vi "JKI.Robot.SMO.TestUI.TestLauncher.vi"() -> ()   [LabVIEW 2014, in "JKI.Robot.SMO.APITesterUI.lvclass"]
doc: "JKI State Machine Objects (SMO) 1.0.0.5\nJKI - JKI\nCopyright (c) 2016, JKI"
uses:
  JKI.Robot.SMO.APITesterUI.lvclass
  <vilib>/JKI/JKI SMO/SMO/SMO.lvclass
  <vilib>/JKI/JKI SMO/SMO.UI/SMO.UI.lvclass
panel:
  out "error out":errorcluster
  in  "Stop":bool
  # "SMO UI Test Launcher"
  # "For instructions on how to use the JKI State Machine Objects, examples and video tutorials, visit:\nhttp://jki.net/state-machine-objects/\n\nJKI State Machine Objects™\nhttp://jki.net/state-machine-objects/\nCopyright (C) 2005-2015, JKI <info@jki.net>\nALL RIGHTS RESERVED"
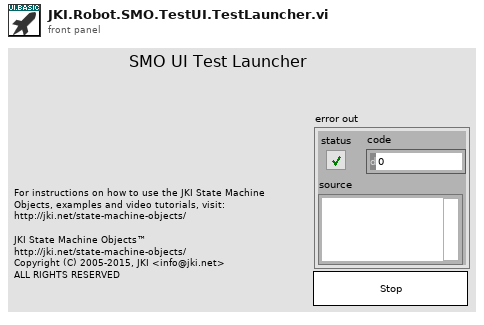
[diagram p1: front panel]
types:
  T1 = typedef "SMO.UI.lvclass/PublicEvents--Cluster.ctl" = cluster{"UI Hidden":refnum<user-event>, "UI State":refnum<user-event>}
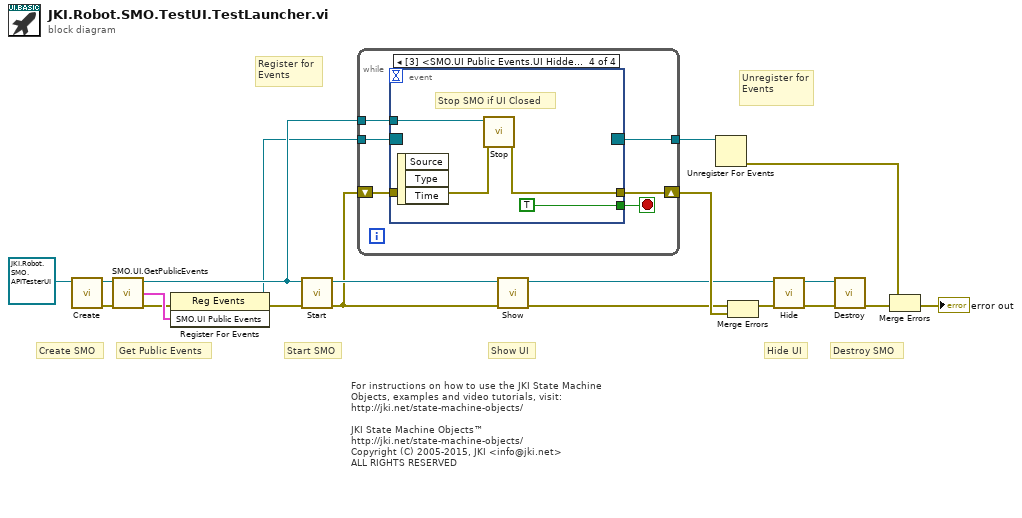
[diagram p0: block diagram]
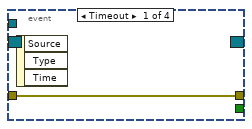
[diagram p2: hidden frame]
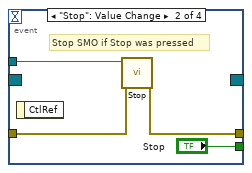
[diagram p3: hidden frame]
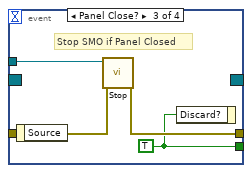
[diagram p4: hidden frame]
diagram:
  # "Hide UI"
  # "Show UI"
  # "For instructions on how to use the JKI State Machine Objects, examples and video tutorials, visit:\nhttp://jki.net/state-machine-objects/\n\nJKI State Machine Objects™\nhttp://jki.net/state-machine-objects/\nCopyright (C) 2005-2015, JKI <info@jki.net>\nALL RIGHTS RESERVED"
  # "Get Public Events"
  # "Start SMO"
  # "Destroy SMO"
  # "Create SMO"
  # "Unregister for Events"
  # "Register for Events"
  n1 = call <vilib>:"Create.vi"("SMO"=refnum<class "JKI.Robot.SMO.APITesterUI.lvclass"> refnum ("SMO.Template.lvclass")) -> ("error out"=w6:errorcluster, "SMO out"=w7:refnum<class "JKI.Robot.SMO.APITesterUI.lvclass">)  [unwired: 8 in, 1 out]
  n2 = call <vilib>:"SMO.UI.GetPublicEvents.vi"("error in (no error)"=w6, "SMO.UI"=w7) -> ("error out"=w3:errorcluster, "SMO.UI Public Events"=w4:T1, "SMO.UI out"=w5:refnum<class "JKI.Robot.SMO.APITesterUI.lvclass">)  [unwired: 7 in]
  n3 = register-events(error in=w3, w4) -> (reference out=w1:refnum<event-registration>, error out=w2:errorcluster)  [unwired: 1 in]
  n4 = call <vilib>:"Start.vi"("error in (no error)"=w2, "SMO"=w5) -> ("error out"=w13:errorcluster, "SMO out"=w14:refnum<class "JKI.Robot.SMO.APITesterUI.lvclass">)  [unwired: 8 in]
  n5 = while {
    shift-right: [w25] -> w19
    shift-left: w13 -> [w24]
    tunnel: w1 -> [w23]
    tunnel: [w22] -> w20
    tunnel: w5 -> [w21]
    stop <- w26 stop-if-true
    n6 = event shown="[3] <SMO.UI Public Events.UI Hidden>: User Event" {
      selector: w23 -> [_ _ _ _]
      dyn-events: [_ _ _ _] -> w22
      timeout: _ -> [_ _ _ _]
      tunnel: [_ "Stop" w32 TRUE ("OK")] -> w26
      tunnel: w21 -> [_ w29 w35 w39]
      tunnel: [w27 w30 w34 w38] -> w25
      tunnel: w24 -> [w27 w28 w33 w37]
      event Timeout {
        n7 = event-data() -> ()  [unwired: 1 in, 3 out]
      }
      event "Stop": Value Change {
        # "Stop SMO if Stop was pressed"
        n8 = event-data() -> ()  [unwired: 1 in, 1 out]
        n9 = call <vilib>:"Stop.vi"("error in (no error)"=w28, "SMO"=w29) -> ("error out"=w30:errorcluster)  [unwired: 8 in, 1 out]
      }
      event Panel Close? {
        w32 = TRUE ("OK")
        # "Stop SMO if Panel Closed"
        n10 = event-data() -> ()  [unwired: 1 in, 1 out]
        n11 = call <vilib>:"Stop.vi"("error in (no error)"=w33, "SMO"=w35) -> ("error out"=w34:errorcluster)  [unwired: 8 in, 1 out]
        n12 = event-data("Discard?"=w32) -> ()  [unwired: 1 in, 1 out]
      }
      event User Event {
        # "Stop SMO if UI Closed"
        n13 = event-data() -> ()  [unwired: 1 in, 3 out]
        n14 = call <vilib>:"Stop.vi"("error in (no error)"=w37, "SMO"=w39) -> ("error out"=w38:errorcluster)  [unwired: 8 in, 1 out]
      }
    }
  }
  n15 = call <vilib>:"Show.vi"("error in (no error)"=w13, "SMO.UI"=w14) -> ("error out"=w12:errorcluster, "SMO.UI out"=w11:refnum<class "JKI.Robot.SMO.APITesterUI.lvclass">)  [unwired: 8 in]
  n16 = Unregister For Events(event registration refnum=w20) -> (error out=w18:errorcluster)  [unwired: 1 in]
  n17 = Merge Errors(w12, w19) -> (w9:errorcluster)
  n18 = call <vilib>:"Hide.vi"("error in (no error)"=w9, "SMO.UI"=w11) -> ("error out"=w8:errorcluster, "SMO.UI out"=w10:refnum<class "JKI.Robot.SMO.APITesterUI.lvclass">)  [unwired: 8 in]
  n19 = call <vilib>:"Destroy.vi"("error in (no error)"=w8, "SMO"=w10) -> ("error out"=w16:errorcluster)  [unwired: 9 in]
  n20 = Merge Errors(w18, w16) -> (→"error out":errorcluster)
